vi "Comm String Wait For ACK.vi"(0 "niDTS Comm Serial in":refnum<class "niDTS Comm Serial.lvclass">, 5 "ACK":string, 7 "Timeout (ms)":i32=1000, 11 "error in (no error)":errorcluster) -> (4 "niDTS Comm Serial out":refnum<class "niDTS Comm Serial.lvclass">, 6 "Response":string, 8 "Sucess":bool, 15 "error out":errorcluster)   [LabVIEW 2015, in "niDTS CommLib.lvlib" / "niDTS Comm Serial.lvclass"]
uses:
  niDTS Comm Serial.lvclass
  String_class/niDTS Comm String.lvclass
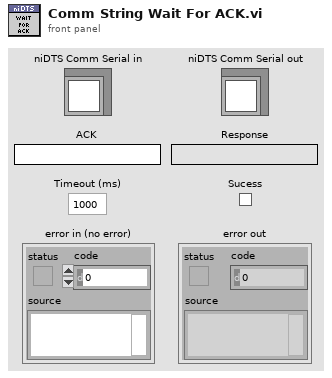
[diagram p1: front panel]
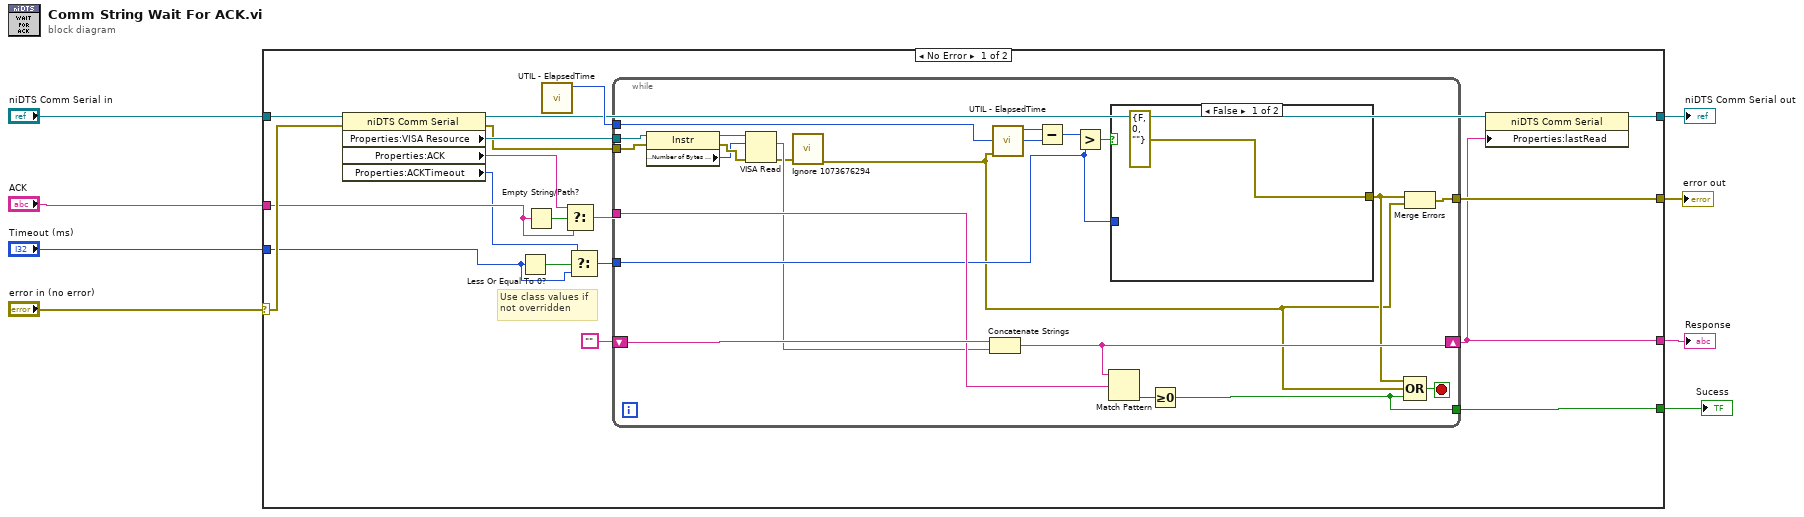
[diagram p0: block diagram]
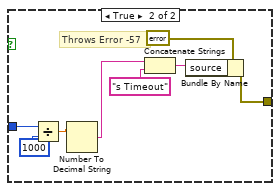
[diagram p2: hidden frame]
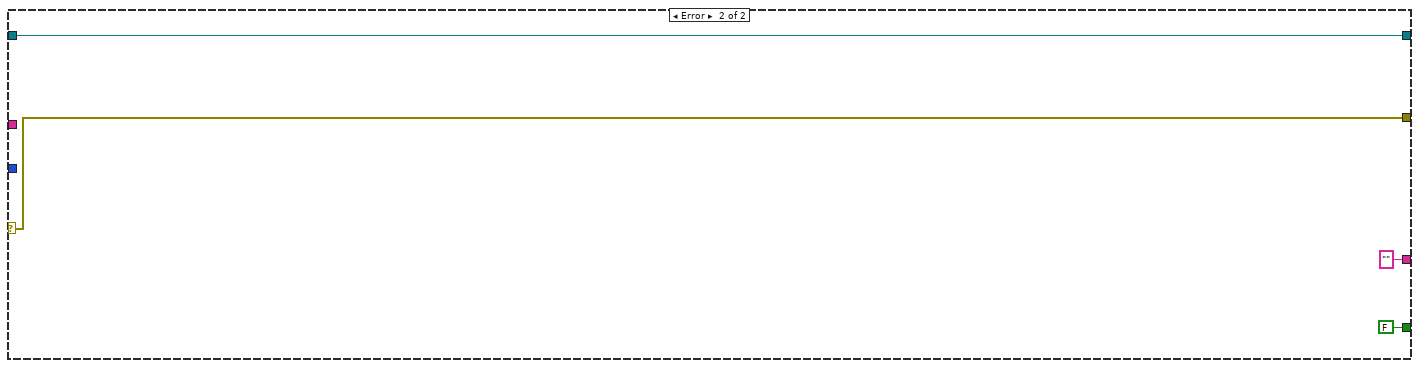
[diagram p3: hidden frame]
diagram:
  n1 = case shown="No Error" "error in (no error)" {
    selector: "error in (no error)" -> [w26 w60]
    tunnel: "niDTS Comm Serial in" -> [w27 w61]
    tunnel: "ACK" -> [w23 _]
    tunnel: "Timeout (ms)" -> [w21 _]
    tunnel: [w13 w61] -> w1
    tunnel: [w12 w60] -> w4
    tunnel: [w11 FALSE] -> w3
    tunnel: [w10 ""] -> w2
    frame No Error {
      # "Use class values if \nnot overridden"
      n2 = property class="niDTS Comm Serial"(reference=w27, error in=w26) -> (reference out=w14:refnum<class "niDTS Comm Serial.lvclass">, error out=w9:errorcluster, "Properties:VISA Resource"=w16:refnum<visa-resource-name>, "Properties:ACK"=w22:string, "Properties:ACKTimeout"=w20:i32)
      n3 = Less Or Equal To 0?(x=w21) -> (x <= 0?=w25:bool)
      n4 = Empty String/Path?(string/path=w23) -> (empty?=w24:bool)
      n5 = call "UTIL - ElapsedTime.vi"() -> ("ms value"=w15:u32)  [unwired: 9 in, 2 out]
      n6 = Select(t=w22, s=w24, f=w23) -> (s? t:f=w18:string)
      n7 = Select(t=w20, s=w25, f=w21) -> (s? t:f=w19:i32)
      n8 = while {
        tunnel: [w39] -> w12
        shift-right: [w46] -> w10
        shift-left: "" -> [w48]
        tunnel: w18 -> [w45]
        tunnel: w15 -> [w42]
        tunnel: w19 -> [w37]
        tunnel: [w36] -> w11
        tunnel: w16 -> [w33]
        tunnel: w9 -> [w28]
        stop <- w44 stop-if-true
        n9 = property class="Instr"(reference=w33, error in=w28) -> (reference out=w29:refnum<visa-resource-name>, error out=w35:errorcluster, "Serial Settings:Number of Bytes at Serial Port"=w34:u32)
        n10 = VISA Read(VISA resource name=w29, byte count=w34, error in (no error)=w35) -> (read buffer=w32:string, error out=w31:errorcluster)  [unwired: 2 out]
        n11 = call "Ignore 1073676294.vi"("error in (no error)"=w31) -> ("error out"=w30:errorcluster)  [unwired: 10 in]
        n12 = Concatenate Strings(w48, w32) -> (w46:string)
        n13 = call "UTIL - ElapsedTime.vi"("error in"=w30) -> ("ms value"=w43:u32)  [unwired: 8 in, 2 out]
        n14 = Subtract(x=w43, y=w42) -> (x-y=w41:u32)
        n15 = Greater?(x=w41, y=w37) -> (0:w40:bool)
        n16 = Match Pattern(string=w46, regular expression=w45) -> (offset past match=w47:i32)  [unwired: 1 in, 3 out]
        n17 = case shown="False" w40 {
          tunnel: [errorcluster {"status"=FALSE, "code"=0, "source"=""} ("error constant") w51] -> w38
          tunnel: w37 -> [_ w57]
          frame False {
          }
          frame True {
            # "Throws Error -57"
            n18 = Divide(x=w57, y=1000) -> (x/y=w55:dbl)
            n19 = Number To Decimal String(number=w55) -> (decimal integer string=w50:string)  [unwired: 1 in]
            n20 = Concatenate Strings(w50, "s Timeout") -> (w52:string)
            n21 = Bundle By Name(cluster=errorcluster {"status"=TRUE, "code"=-57, "source"="40 s Timeout"} ("error constant"), "source"=w52) -> (w51:errorcluster)
          }
        }
        n22 = Greater Or Equal To 0?(x=w47) -> (x >= 0?=w36:bool)
        n23 = Compound Arithmetic op=OR(w38, w30, w36) -> (w44:bool)
        n24 = Merge Errors(w38, w30) -> (w39:errorcluster)
      }
      n25 = property class="niDTS Comm Serial"(reference=w14, "Properties:lastRead"=w10) -> (reference out=w13:refnum<class "niDTS Comm Serial.lvclass">)  [unwired: 1 in, 1 out]
    }
    frame Error {
    }
  }
  "error out" <- w4
  "niDTS Comm Serial out" <- w1
  "Response" <- w2
  "Sucess" <- w3
